vi "Read Revision.vi"(8 "error in":errorcluster, 11 "Engine in":refnum<class "Engine.lvclass">) -> (0 "error out":errorcluster, 2 "Version":string, 3 "Engine out":refnum<class "Engine.lvclass">)   [LabVIEW 2023, in "Engine.lvlib" / "Engine.lvclass"]
uses:
  Project/Engine.lvclass
  Project/Engine.lvclass/Engine.ctl
  <vilib>/Utility/error.llb/Error Cluster From Error Code.vi
  <vilib>/ErrorRing/Error Ring.xnode
  <vilib>/Utility/LVLibp/NI_PackedLibraryUtility.lvlib
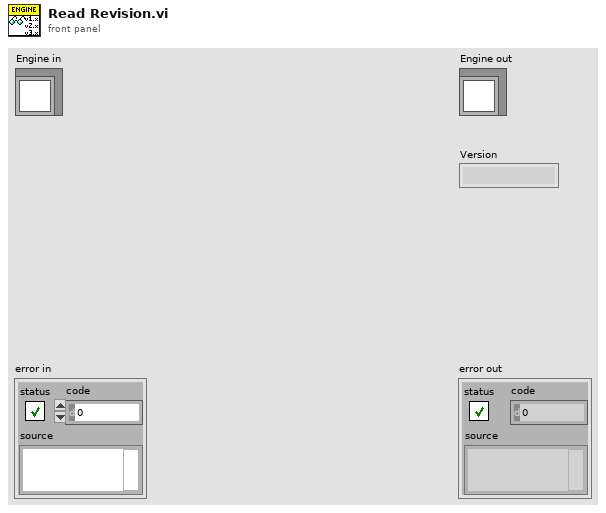
[diagram p1: front panel]
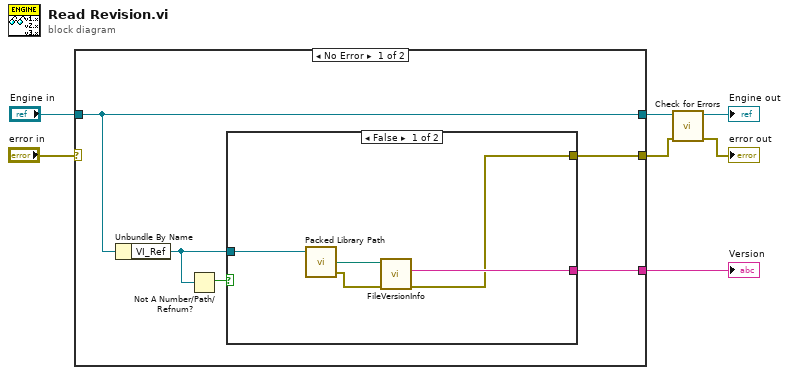
[diagram p0: block diagram]
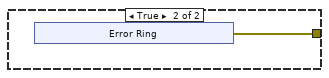
[diagram p2: hidden frame]
diagram:
  n1 = case shown="No Error" "error in" {
    selector: "error in" -> [_ w24]
    tunnel: [w12 _] -> w7
    tunnel: "Engine in" -> [w9 w23]
    tunnel: [w9 w23] -> w4
    tunnel: [w8 w24] -> w2
    frame No Error {
      n2 = Unbundle By Name(w9) -> ("VI_Ref"=w11:refnum<vi>)
      n3 = Not A Number/Path/Refnum?(number/path/refnum=w11) -> (NaN/Path/Refnum?=w10:bool)
      n4 = case shown="False" w10 {
        tunnel: [w15 _] -> w12
        tunnel: w11 -> [w17 _]
        tunnel: [w13 w18] -> w8
        frame False {
          n5 = call <vilib>:"Packed Library Path.vi"("vi reference"=w17) -> ("error out"=w14:errorcluster, "packed library path"=w16:path)  [unwired: 2 in, 1 out]
          n6 = call <vilib>:"FileVersionInfo.vi"("error in (no error)"=w14, "Application Path in"=w16) -> ("error out"=w13:errorcluster, "File Version Info"=w15:string)  [unwired: 6 in, 2 out]
        }
        frame True {
          n7 = xnode "Error Ring"() -> ("error out"=w18:errorcluster)
        }
      }
    }
    frame Error {
    }
  }
  "Version" <- w7
  n8 = call "Check for Errors.vi"("error in"=w2, "Engine in"=w4) -> ("error out"=→"error out":errorcluster, "Engine out"=→"Engine out":refnum<class "Engine.lvclass">)  [unwired: 8 in]
